vi "U64 Timer Global.vi"() -> ()   [LabVIEW 2024]
panel:
  in  "Stop Tick Count (U64)":bool
  in  "Tick Count (U64)":u64
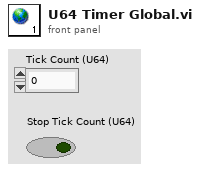
[diagram p1: front panel]
diagram:
